vi "Exponential.vi"() -> ()   [LabVIEW 2023]
doc: "This example shows how the Exponential function operates with different data types. These concepts also apply to the Exponential (Arg) -1, Power Of 10, Power Of 2, Power Of X, Y-th Root of X, Natural Logarithm, Natural Logarithm (Arg +1), Logarithm Base 10, Logarithm Base 2, and Logarithm Base X functions."
panel:
  in  "Tab Control":T1(tab)
  out "exp(x)":dbl=1.0
  in  "numeric":dbl
  out "exp(x)":dbl[](array[numeric])
  in  "Array":dbl[](array[numeric])=[0.0, 1.0, 2.0, 3.0, 4.0]
  out "exp(x)":cluster{"numeric 1":dbl, "numeric 2":dbl}
  in  "Cluster":cluster{"numeric 1":dbl, "numeric 2":dbl}={"numeric 1"=0.0, "numeric 2"=1.0}
  out "exp(x)":cluster{"numeric 1":dbl, "numeric 2":dbl}[](array[cluster])
  in  "Array of Cluster":cluster{"numeric 1":dbl, "numeric 2":dbl}[](array[cluster])=[{"numeric 1"=0.0, "numeric 2"=1.0}, {"numeric 1"=2.0, "numeric 2"=3.0}, {"numeric 1"=4.0, "numeric 2"=5.0}]
  # "Overview: Demonstrates how the Exponential function operates with different data types.\nInstructions:\n1. Run the VI.\n2. Examine the different cases.\n3. Although this example demonstrates the Exponential function, the concepts also apply to other Exponential Functions."
  # "The exponential of the numeric is computed to give exp(x)."
  # "The exponential of each element in the array is computed to give an array of exp(x)."
  # "The exponential of each element in the cluster is computed to give a cluster of exp(x).  A cluster of numeric arrays would produce a cluster of numeric arrays."
  # "The exponential of each element in the array is computed to give an array of clusters of exp(x)."
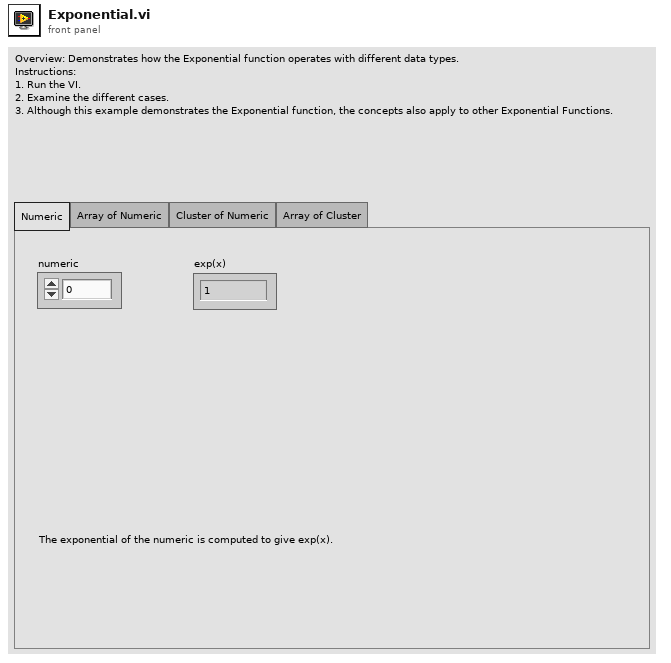
[diagram p1: front panel]
types:
  T1 = enum32{"Numeric", "Array of Numeric", "Cluster of Numeric", "Array of Cluster"}
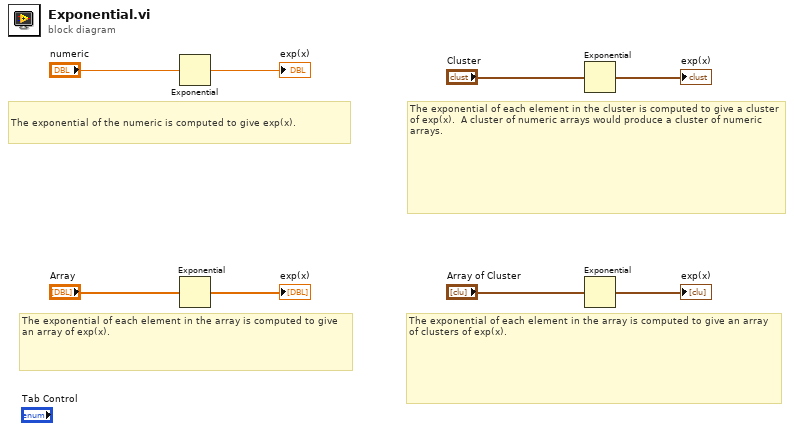
[diagram p0: block diagram]
diagram:
  # "The exponential of each element in the array is computed to give an array of clusters of exp(x)."
  # "The exponential of each element in the cluster is computed to give a cluster of exp(x).  A cluster of numeric arrays would produce a cluster of numeric arrays."
  # "The exponential of each element in the array is computed to give an array of exp(x)."
  # "The exponential of the numeric is computed to give exp(x)."
  n1 = Exponential(1:"numeric") -> (0:→"exp(x)":dbl)
  n2 = Exponential(1:"Array") -> (0:→"exp(x)":dbl[])
  n3 = Exponential(1:"Cluster") -> (0:→"exp(x)":cluster{"numeric 1":dbl, "numeric 2":dbl})
  n4 = Exponential(1:"Array of Cluster") -> (0:→"exp(x)":cluster{"numeric 1":dbl, "numeric 2":dbl}[])
